vi "Teleop.vi"(10 "Match Info":T2={"Autonomous Elapsed Seconds"=0.0, "TeleOp Elapsed Seconds"=0.0, "Disabled Elapsed Seconds"=0.0, "Visited Autonomous"=FALSE, "Visited TeleOp"=FALSE, "Visited Disabled"=FALSE, "Autonomous Settings"={"Autonomous Style"=enum."Independent", "VI Refnum"=refnum}}, 11 "Call Context":T3) -> ()   [LabVIEW 2018]
doc: "This VI is called for each TeleOp packet received from the DS where the robot is not disabled. It is often used to read from the joysticks and update I/O or to update setpoints for timed control loops. It should complete and return within 20 milliseconds or it may miss DS packets."
uses:
  <vilib>/Rock Robotics/WPI/DriverStation/WPI_DriverStationDerivedRobotMode.ctl
  <vilib>/Rock Robotics/WPI/DriverStation/WPI_DriverStationMatch Info.ctl
  TypeDefs/Teleop Data Cluster.ctl
  TypeDefs/typedef_enum_Teleop.ctl
  TypeDefs/typedef_enum_Refnums.ctl
  TypeDefs/Joystick Buttons.ctl
  TypeDefs/Joystick Axes.ctl
  <vilib>/Rock Robotics/Network Tables/NT Write Boolean.vi
panel:
  in  "drive b":dbl=0.05 format="%#_13g"
  in  "drive fast a":dbl=0.9 format="%#_13g"
  in  "drive a":dbl=0.8 format="%#_13g"
  in  "lower limit":dbl=-0.8 format="%#_13g"
  in  "upper limit":dbl=0.8 format="%#_13g"
  in  "Cluster 2":T1
  out "Loop Time":u32
  in  "joystick lower limit":dbl=-0.5 format="%#_13g"
  in  "joystick upper limit":dbl=0.5 format="%#_13g"
  in  "joystick scale factor":dbl=0.5
  out "notifier out":refnum<notifier>
  in  "Cluster":T1
  out "error out":errorcluster
  in  "error in":errorcluster
  # "wrist stuff!! used to be +- .4"
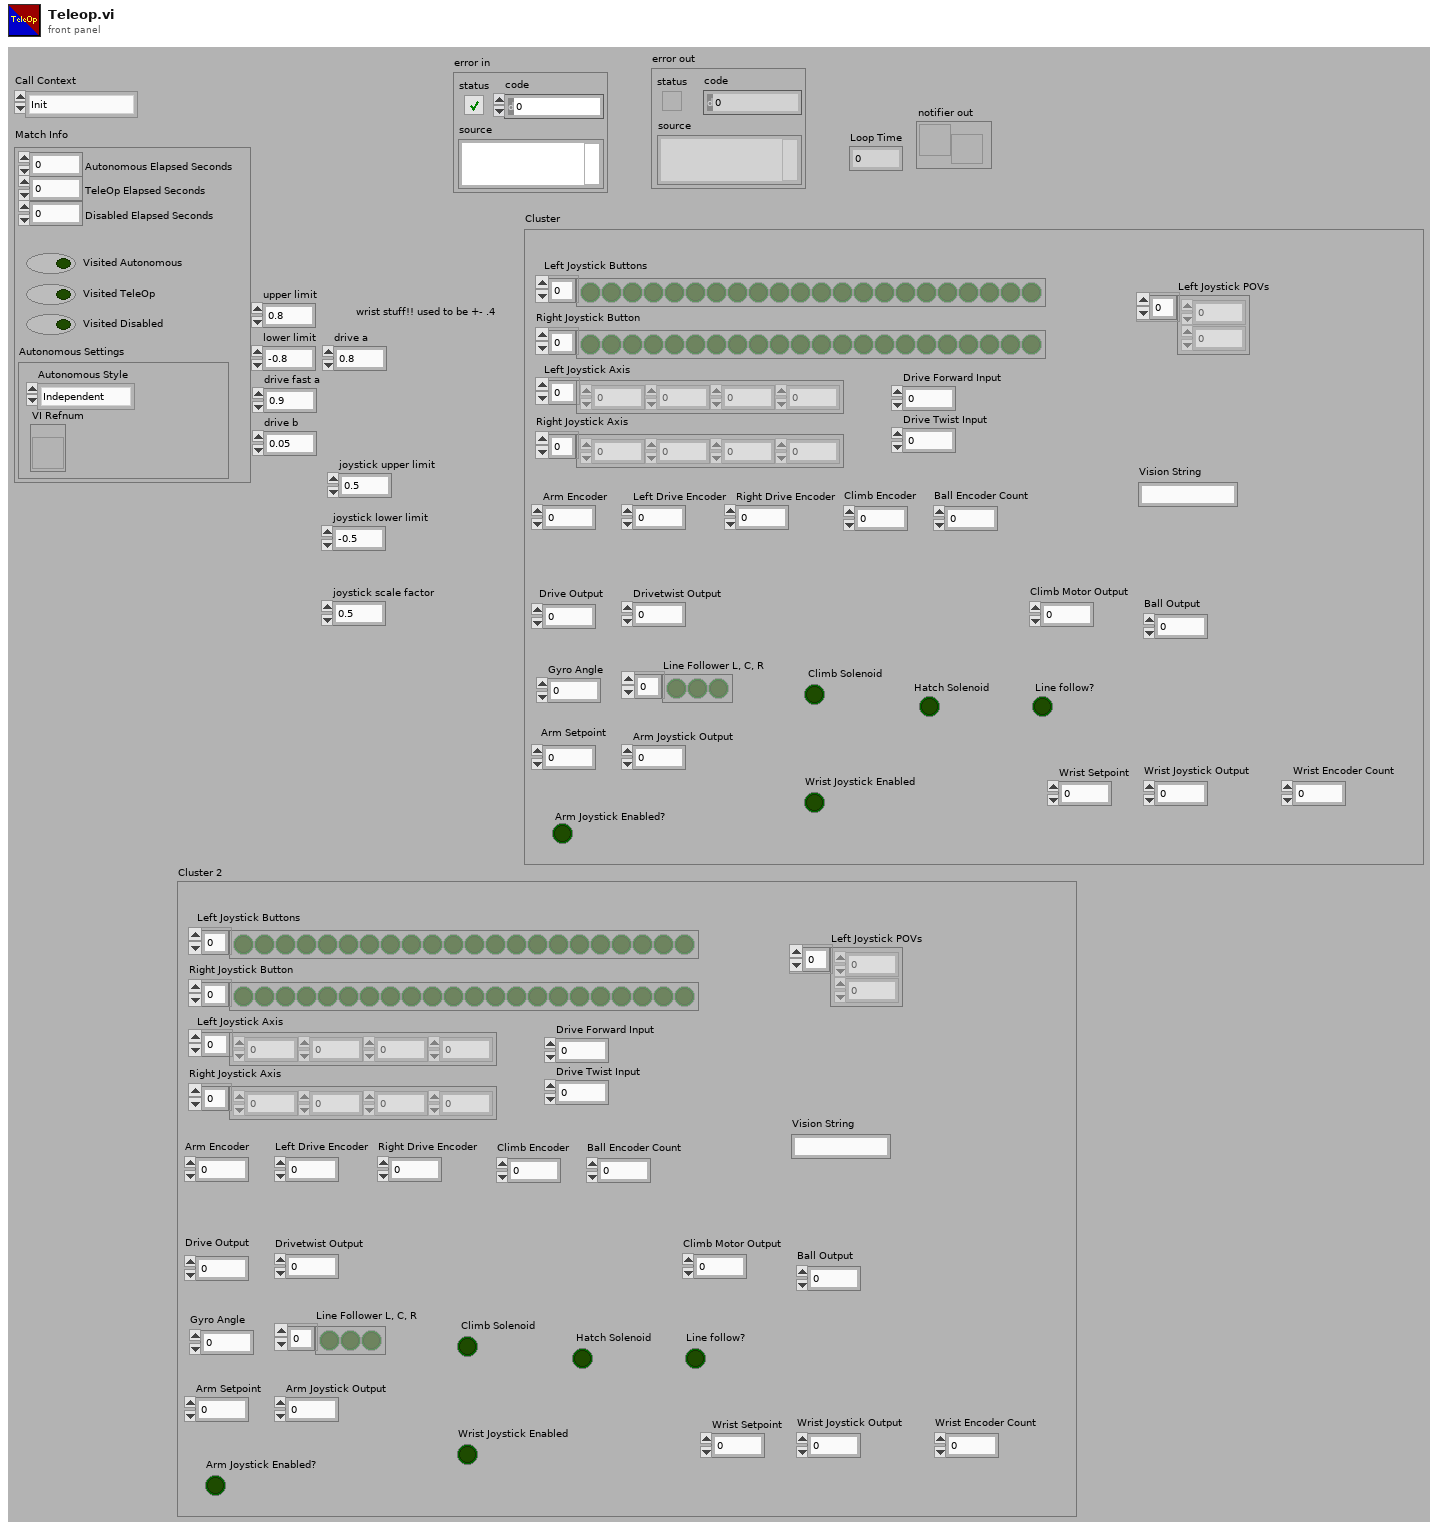
[diagram p1: front panel]
types:
  T1 = typedef "Teleop Data Cluster.ctl" = cluster{"Drive Forward Input ":dbl, "Drive Twist Input":dbl, "Drive Output":dbl, "Drivetwist Output":dbl, "Left Joystick Buttons":bool[], "Left Joystick Axis":dbl[], "Right Joystick Axis":dbl[], "Right Joystick Button":bool[], "Arm Encoder":dbl, "Left Drive Encoder":dbl, "Right Drive Encoder":dbl, "Gyro Angle ":dbl, "Arm Joystick Output  ":dbl, "Line Follower L, C, R ":bool[], "Line follow?":bool, " Climb Solenoid":bool, "Wrist Encoder Count":dbl, "Wrist Joystick Output":dbl, "Ball Encoder Count":dbl, "Ball Output":dbl, "Climb Encoder":dbl, "Climb Motor Output":dbl, " Hatch Solenoid":bool, "Arm Setpoint ":dbl, "Wrist Setpoint ":dbl, "Arm Joystick Enabled?":bool, "Wrist Joystick Enabled":bool, "Vision String":string, "Left Joystick POVs":i16[]}
  T2 = typedef "WPI_DriverStationMatch Info.ctl" = cluster{"Autonomous Elapsed Seconds":dbl, "TeleOp Elapsed Seconds":dbl, "Disabled Elapsed Seconds":dbl, "Visited Autonomous":bool, "Visited TeleOp":bool, "Visited Disabled":bool, "Autonomous Settings":cluster{"Autonomous Style":enum16{"Iterative", "Independent"}, "VI Refnum":refnum<vi>}}
  T3 = typedef "WPI_DriverStationDerivedRobotMode.ctl" = enum16{"Init", "Execute", "Stop"}
  T4 = typedef "typedef_enum_Refnums.ctl" = enum16{"Ball_Encoder", "Ball_Motor", "Camera", "Linefollow_3", "Linefollow_2", "Linefollow_1", "Gyro", "Hatch_Solenoid", "Climb_Back_Solenoid", "Arm_Encoder", "Arm_Motor", "Lift_Encoder", "Drive", "Drive_Motor_R", "Drive_Motor_L", "Drive_Encoder_R", "Drive_Encoder_L", "Joy_R", "Joy_L", "Wrist_Motor", "Wrist_Encoder", "Climb Upper Limit", "Climb Lower Limit ", "Climb_Front_Motor"}
  T5 = typedef "typedef_enum_Teleop.ctl" = enum16{"Wait", "Drive_Forward", "Drive_Turn", "Arm", "Wrist", "Intake", "Climb", "Gyro", "Line Follower", "Vision_Calculations", "Send_Notifier"}
  T6 = typedef "Joystick Buttons.ctl" = enum16{"Trigger", "Thumb", "Top 3", "Top 4", "Top 5", "Top 6", "Bottom 7", "Bottom 8", "Bottom 9", "Bottom 10", "Bottom 11", "Bottom 12"}
  T7 = typedef "Joystick Axes.ctl" = enum16{"X Axis", "Y Axis", "Twist Axis", "Throttle"}
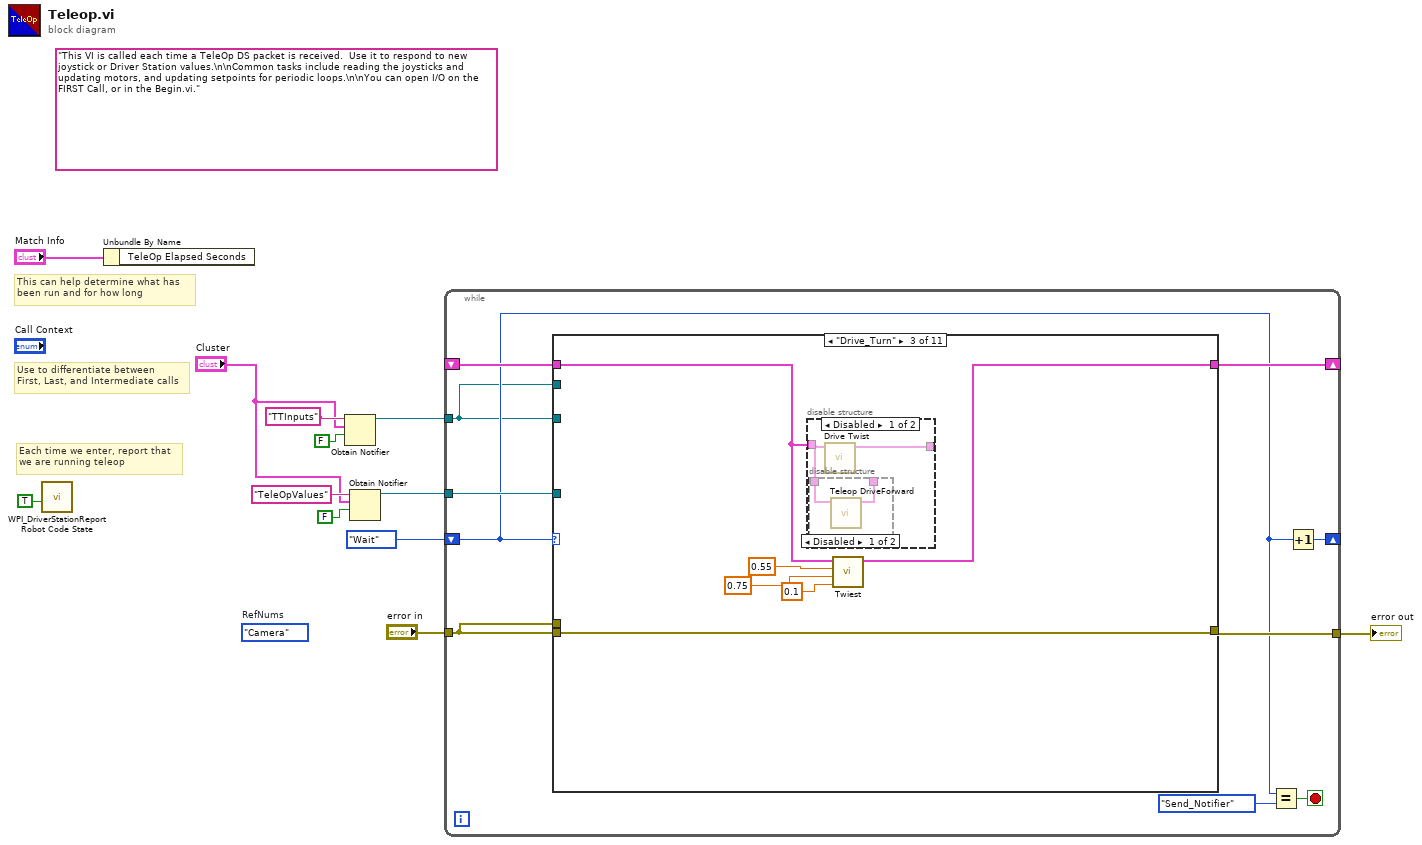
[diagram p0: block diagram]
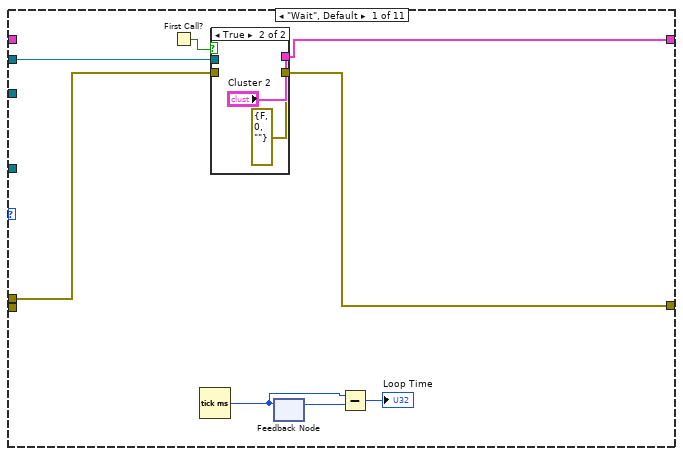
[diagram p2: hidden frame]
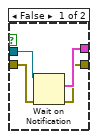
[diagram p3: hidden frame]
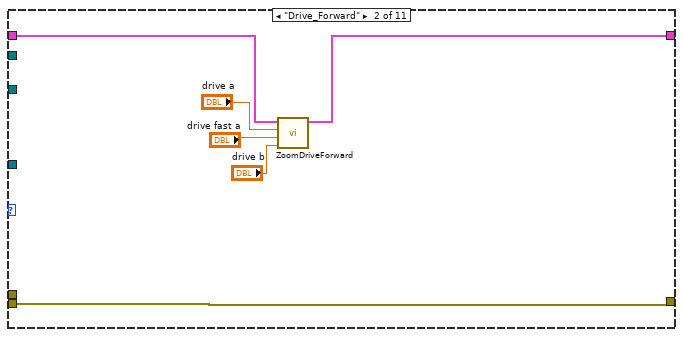
[diagram p4: hidden frame]
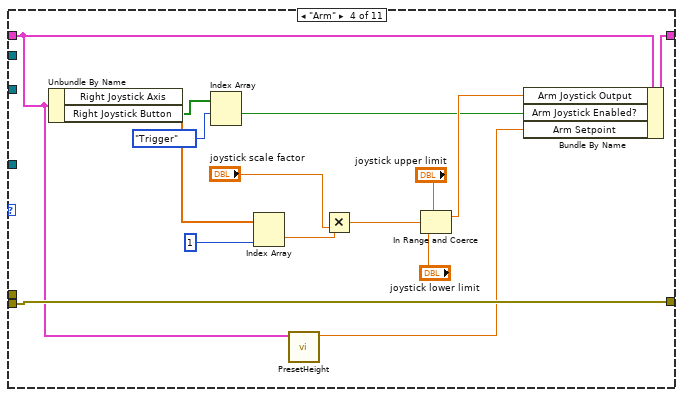
[diagram p7: hidden frame]
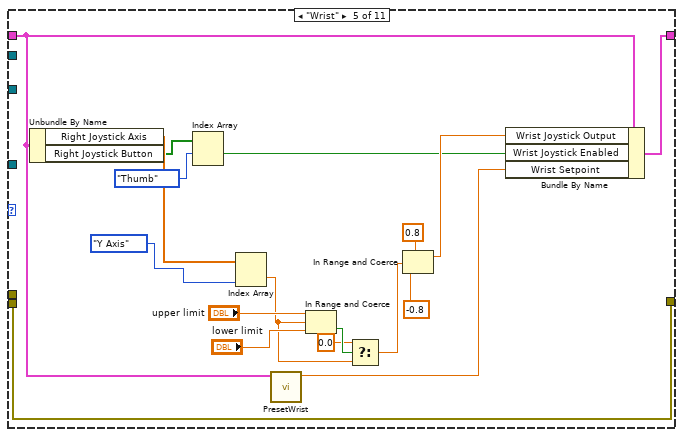
[diagram p8: hidden frame]
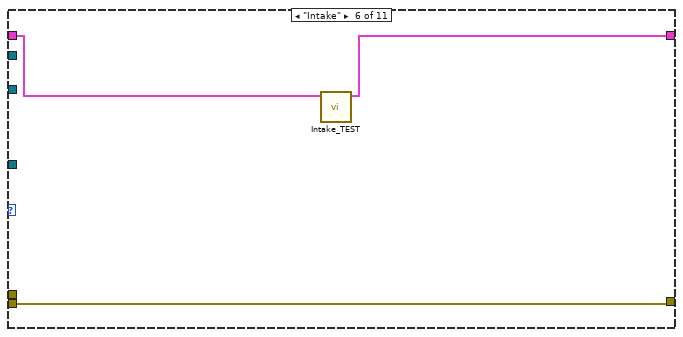
[diagram p9: hidden frame]
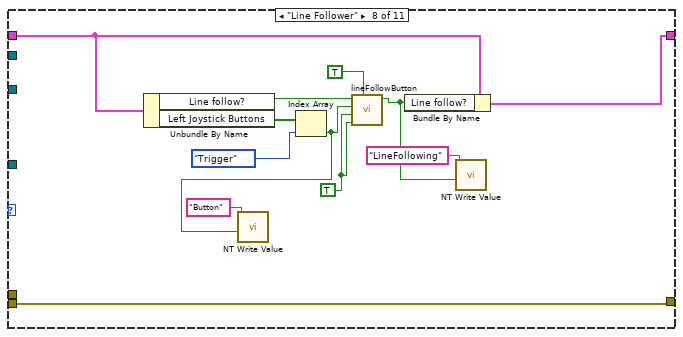
[diagram p11: hidden frame]
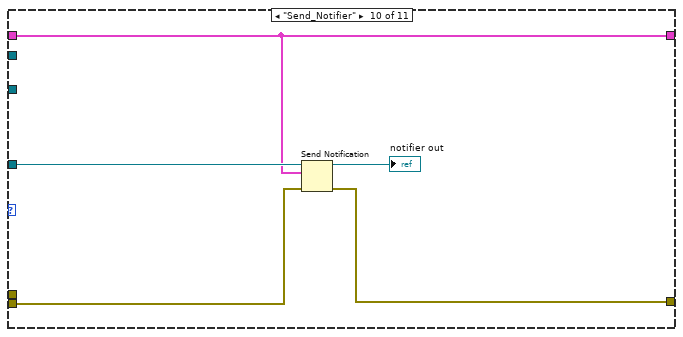
[diagram p13: hidden frame]
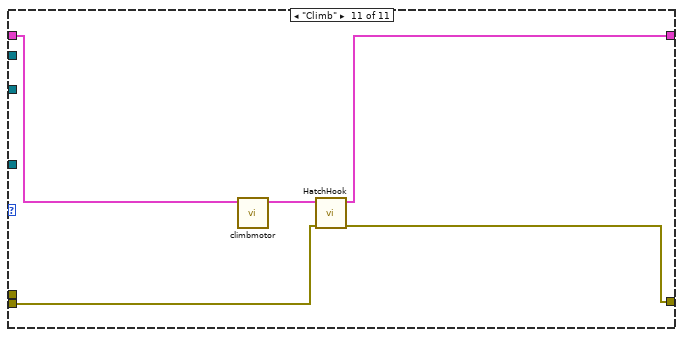
[diagram p14: hidden frame]
diagram:
  (unwired) typedef_enum_Refnums."Camera"  # RefNums
  (unwired) "This VI is called each time a TeleOp DS packet is received.  Use it to respond to new joystick or Driver Station values.\n\nCommon tasks include reading the joysticks and updating motors, and updating setpoints for periodic loops.\n\nYou can open I/O on the FIRST Call, or in the Begin.vi."
  # "Each time we enter, report that\nwe are running teleop"
  # "Use to differentiate between\nFirst, Last, and Intermediate calls"
  # "This can help determine what has\nbeen run and for how long"
  n1 = call <vilib>:"WPI_DriverStationReport Robot Code State.vi"("TeleOp"=TRUE ("Autonomous")) -> ()  [unwired: 10 in, 1 out]
  n2 = Unbundle By Name("Match Info") -> ()  [unwired: 1 out]
  n3 = Obtain Notifier(name (unnamed)="TTInputs", notification data type="Cluster", create if not found? (T)=FALSE) -> (notifier out=w8:refnum<notifier>)  [unwired: 1 in, 2 out]
  n4 = Obtain Notifier(name (unnamed)="TeleOpValues", notification data type="Cluster", create if not found? (T)=FALSE) -> (notifier out=w7:refnum<notifier>)  [unwired: 1 in, 2 out]
  n5 = while {
    tunnel: w8 -> [w14]
    tunnel: w7 -> [w22]
    shift-right: [w21] -> _
    shift-left: typedef_enum_Teleop."Wait" ("Enum") -> [w15]
    tunnel: [w20] -> w3
    tunnel: "error in" -> [w13]
    shift-right: [w19] -> _
    shift-left: _ -> [w18]
    stop <- w17 stop-if-true
    n6 = case shown="\"Drive_Turn\"" w15 {
      tunnel: w14 -> [_ _ _ _ _ _ _ _ _ _ _]
      tunnel: w22 -> [_ _ _ _ _ _ _ _ _ w109 _]
      tunnel: [w23 w40 w48 w67 w85 w86 w89 w102 w103 w107 w113] -> w20
      tunnel: w13 -> [_ w40 w48 w67 w85 w86 w89 w102 w103 w108 w112]
      tunnel: [w24 w41 w43 w54 w75 w87 w90 w100 w104 w106 w114] -> w19
      tunnel: w18 -> [_ w42 w47 w55 w76 w88 w90 w99 w104 w106 w111]
      tunnel: w14 -> [w26 _ _ _ _ _ _ _ _ _ _]
      tunnel: w13 -> [w25 _ _ _ _ _ _ _ _ _ _]
      frame "Wait", Default {
        n7 = First Call?() -> (First Call?: T/F=w27:bool)
        n8 = Tick Count (ms)() -> (millisecond timer value=w29:u32)
        n9 = case shown="True" w27 {
          tunnel: w26 -> [w34 _]
          tunnel: w25 -> [w33 _]
          tunnel: [w32 "Cluster 2"] -> w24
          tunnel: [w31 errorcluster {"status"=FALSE, "code"=0, "source"=""} ("error out")] -> w23
          frame False {
            n10 = Wait on Notification(notifier=w34, error in (no error)=w33) -> (notification=w32:T1, error out=w31:errorcluster)  [unwired: 2 in, 2 out]
          }
          frame True {
          }
        }
        n11 = feedback-in #1(w29) -> ()
        n12 = feedback #1() -> (w30:u32)  [unwired: 1 in]
        n13 = Subtract(x=w29, y=w30) -> (x-y=→"Loop Time":u32)
      }
      frame "Drive_Forward" {
        n14 = call "ZoomDriveForward.vi"("b Value"="drive b", "fastvalue"="drive fast a", "Mormal Value"="drive a", "Cluster In"=w42) -> ("Cluster Out"=w41:T1)  [unwired: 7 in]
      }
      frame "Drive_Turn" {
        n15 = disable-structure shown="Disabled" {
          disable-tunnel: w47 -> [w50 _]
          disable-tunnel: [w49 _] -> _
          frame Disabled {
            n16 = disable-structure shown="Disabled" {
              disable-tunnel: w50 -> [w52 _]
              disable-tunnel: [w51 _] -> _
              frame Disabled {
                n17 = call "Teleop DriveForward.vi"("Data Input"=w52) -> ("Data Output"=w51:T1)  [unwired: 9 in, 1 out]
              }
              frame Enabled {
              }
            }
            n18 = call "Drive Twist.vi"("Cluster"=w50) -> ("Cluster 2"=w49:T1)  [unwired: 10 in]
          }
          frame Enabled {
          }
        }
        n19 = call "Twiest.vi"("b Value"=0.1, "fastvalue"=0.75, "Mormal Value"=0.55, "Cluster In"=w47) -> ("Cluster Out"=w43:T1)  [unwired: 7 in]
      }
      frame "Arm" {
        n20 = Unbundle By Name(w55) -> ("Right Joystick Axis"=w66:dbl[], "Right Joystick Button"=w58:bool[])
        n21 = Index Array(array=w58, index #1=Joystick_Buttons."Trigger" ("Enum")) -> (element #1=w56:bool)  [unwired: 1 in, 1 out]
        n22 = Index Array(array=w66, index #2=1 ("index")) -> (element #2=w60:dbl)  [unwired: 1 in, 1 out]
        n23 = call "PresetHeight.vi"("Cluster"=w55) -> ("Numeric"=w53:dbl)  [unwired: 10 in]
        n24 = Multiply(x=w60, y="joystick scale factor") -> (x*y=w63:dbl)
        n25 = In Range and Coerce(upper limit="joystick upper limit", x=w63, lower limit="joystick lower limit") -> (coerced(x)=w65:dbl)  [unwired: 1 out]
        n26 = Bundle By Name(cluster=w55, "Arm Joystick Output"=w65, "Arm Joystick Enabled?"=w56, "Arm Setpoint"=w53) -> (w54:T1)
      }
      frame "Wrist" {
        n27 = Unbundle By Name(w76) -> ("Right Joystick Axis"=w84:dbl[], "Right Joystick Button"=w80:bool[])
        n28 = Index Array(array=w80, index #1=Joystick_Buttons."Thumb" ("Enum")) -> (element #1=w78:bool)  [unwired: 1 in, 1 out]
        n29 = Index Array(array=w84, index #2=Joystick_Axes."Y Axis" ("Enum")) -> (element #2=w69:dbl)  [unwired: 1 in, 1 out]
        n30 = call "PresetWrist.vi"("Cluster"=w76) -> ("Numeric"=w77:dbl)  [unwired: 10 in]
        n31 = In Range and Coerce(upper limit="upper limit", x=w69, lower limit="lower limit") -> (In Range?=w71:bool)  [unwired: 1 out]
        n32 = Select(t=0.0, s=w71, f=w69) -> (s? t:f=w68:dbl)
        n33 = In Range and Coerce(upper limit=0.8 ("joystick upper limit 2"), x=w68, lower limit=-0.8 ("joystick lower limit 2")) -> (coerced(x)=w83:dbl)  [unwired: 1 out]
        n34 = Bundle By Name(cluster=w76, "Wrist Joystick Output"=w83, "Wrist Joystick Enabled"=w78, "Wrist Setpoint"=w77) -> (w75:T1)
      }
      frame "Intake" {
        n35 = call "Intake_TEST.vi"("CLUSTERIN"=w88) -> ("ClusterOUT"=w87:T1)  [unwired: 10 in]
      }
      frame "Gyro" {
      }
      frame "Line Follower" {
        w95 = TRUE ("Left")
        n36 = Unbundle By Name(w99) -> ("Line follow?"=w101:bool, "Left Joystick Buttons"=w98:bool[])
        n37 = Index Array(array=w98, index=Joystick_Buttons."Trigger" ("Enum")) -> (element=w91:bool)
        n38 = call-poly <vilib>:"NT Write Value.vi"("Boolean"=w91, "Name"="Button") -> ()  [unwired: 9 in, 1 out]
        n39 = call "lineFollowButton.vi"("Right"=TRUE, "Middle"=w95, "Left"=w95, "Line Following Button"=w91, "Currently Line Following?"=w101) -> ("Still Line Following?"=w94:bool)  [unwired: 6 in]
        n40 = Bundle By Name(cluster=w99, "Line follow?"=w94) -> (w100:T1)
        n41 = call-poly <vilib>:"NT Write Value.vi"("Boolean"=w94, "Name"="LineFollowing") -> ()  [unwired: 9 in, 1 out]
      }
      frame "Vision_Calculations" {
      }
      frame "Send_Notifier" {
        n42 = Send Notification(notification=w106, notifier=w109, error in (no error)=w108) -> (notifier out=→"notifier out":refnum<notifier>, error out=w107:errorcluster)
      }
      frame "Climb" {
        n43 = call "climbmotor.vi"("Cluster 2"=w111) -> ("Cluster"=w110:T1)  [unwired: 9 in]
        n44 = call "HatchHook.vi"("error in"=w112, "ClusterIN"=w110) -> ("error out"=w113:errorcluster, "ClusterOUT"=w114:T1)  [unwired: 8 in]
      }
    }
    n45 = Equal?(x=w15, y=typedef_enum_Teleop."Send_Notifier" ("Enum")) -> (x = y?=w17:bool)
    n46 = Increment(x=w15) -> (x+1=w21:T5)
  }
  "error out" <- w3
